vi "ArmKinematicsSimulator.vi"() -> ()   [LabVIEW 2020]
doc: "Simulates the inverse and forward kinematics for the configured robot arm on the computer, without needing to deploy to the robot."
uses:
  <vilib>/Utility/miscctls.llb/LV3DPointTypeDef.ctl
  GlobalArm.vi
  <vilib>/picture/3D Picture Control/Object/Create Object (drawable).vi
  <vilib>/picture/3D Picture Control/Object/Add Object (no reference).vi
  <vilib>/picture/3D Picture Control/NI_3D Picture Control.lvlib
  <vilib>/robotics/Kinematics/Plotting/NI_Robotics_3DKinematics.lvlib
panel:
  out "Wrist Power [-1, 1]":dbl format="%.2f"
  out "Elbow Power [-1. 1]":dbl format="%.2f"
  out "Shoulder Power [-1, 1]":dbl format="%.2f"
  in  "Intial Joint Angle Guesses (deg)":cluster{dbl, dbl, dbl}={90.0, 135.0, 0.0}
  in  "Goal End Effector Position":cluster{dbl, dbl, dbl}={180.0, -30.0, 25.0}
  in  "Reset 3D View":bool
  out "3D Arm Simulation":refnum<vi>(3d-picture)
  # "Pitch (deg)"
  # "X (in)"
  # "Z (in)"
  # "Shoulder (deg)"
  # "Elbow (deg)"
  # "Wrist (deg)"
  # "<-- DOWN FIELD              SCORING GRID -->"
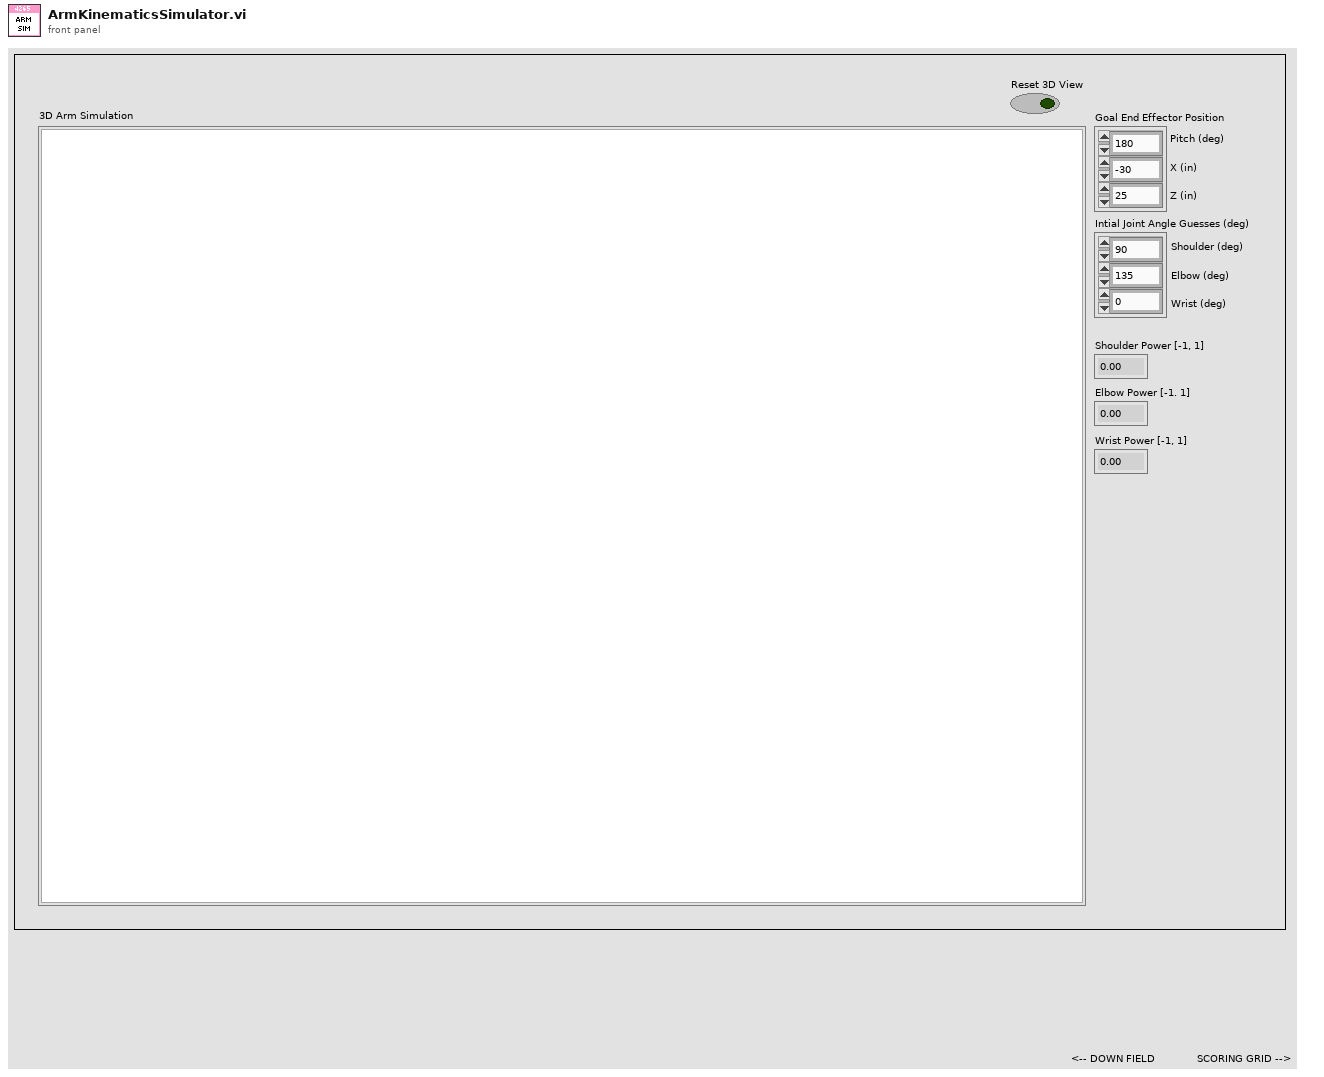
[diagram p1: front panel]
types:
  T1 = cluster{"Red":sgl, "Green":sgl, "Blue":sgl, "Alpha":sgl}
  T2 = typedef "LV3DPointTypeDef.ctl" = cluster{"X":sgl, "Y":sgl, "Z":sgl}
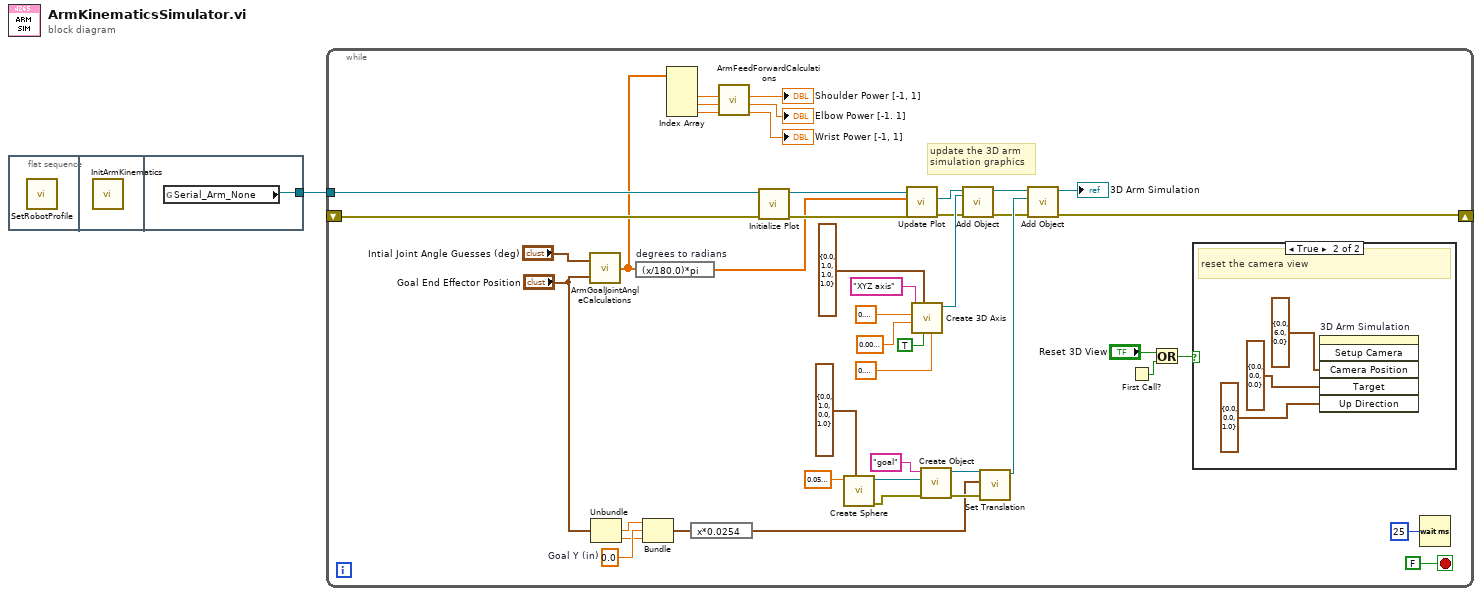
[diagram p0: block diagram]
diagram:
  n1 = flat-sequence {
    tunnel: [w2] -> w1
    frame #0 {
      n2 = call "SetRobotProfile.vi"() -> ()  [unwired: 1 in]
    }
    frame #1 {
      n3 = call "InitArmKinematics.vi"() -> ()  [unwired: 1 in]
    }
    frame #2 {
      n4 = global read "GlobalArm.vi" "Serial_Arm_None"() -> (w2:refnum<class "NI_Robotics_Serial Robot Arm.lvclass">)
    }
  }
  n5 = while {
    tunnel: w1 -> [w31]
    shift-right: [w22] -> _
    shift-left: _ -> [w30]
    stop <- FALSE stop-if-true
    w20 = 0.0  # Goal Y (in)
    # "update the 3D arm\nsimulation graphics"
    n6 = call "ArmGoalJointAngleCalculations.vi"("Goal End Effector Position"="Goal End Effector Position", "Intial Joint Angle Guesses (deg)"="Intial Joint Angle Guesses (deg)") -> ("Goal Joint Angles (deg)"=w9:dbl[])
    n7 = Unbundle("Goal End Effector Position") -> (w14:dbl, w13:dbl)  [unwired: 1 out]
    n8 = expression code="(x/180.0)*pi" "degrees to radians"(w9) -> (w16:dbl[])
    n9 = Bundle(w14, "Goal Y (in)"=w20, w13) -> (w19:cluster{dbl, "Goal Y (in)":dbl, dbl})  [unwired: 1 in]
    n10 = Index Array(array=w9) -> (element #2=w8:dbl, element #3=w7:dbl, element #4=w6:dbl)  [unwired: 4 in, 1 out]
    n11 = expression code="x*0.0254" ("degrees to radians")(w19) -> (w18:cluster{dbl, "Goal Y (in)":dbl, dbl})
    n12 = call "ArmFeedForwardCalculations.vi"("Wrist Pos (deg)"=w6, "Elbow Pos (deg)"=w7, "Shoulder Pos (deg)"=w8) -> ("Wrist Power [-1, 1]"=→"Wrist Power [-1, 1]":dbl, "Elbow Power [-1. 1]"=→"Elbow Power [-1. 1]":dbl, "Shoulder Power [-1, 1]"=→"Shoulder Power [-1, 1]":dbl)  [unwired: 6 in]
    n13 = call <vilib>:"Initialize Plot.vi"("error in (no error)"=w30, "serial arm in"=w31) -> ("error out"=w26:errorcluster, "serial arm out"=w25:refnum<class "NI_Robotics_Serial Robot Arm.lvclass">)  [unwired: 8 in]
    n14 = call <vilib>:"Create Sphere.vi"("Color"=T1 {"Red"=0.0, "Green"=1.0, "Blue"=0.0, "Alpha"=1.0}, "Radius"=sgl 0.05) -> ("error out"=w21:errorcluster, "New Sphere Refnum"=w27:refnum<vi>)  [unwired: 8 in]
    n15 = call <vilib>:"Update Plot.vi"("error in (no error)"=w26, "joint positions"=w16, "serial arm in"=w25) -> ("error out"=w24:errorcluster, "serial arm scene"=w45:refnum<vi>)  [unwired: 6 in, 1 out]
    n16 = call <vilib>:"Create 3D Axis.vi"("Character Size"=sgl 0.1, "Axis label?"=TRUE, "Color"=T1 {"Red"=0.0, "Green"=1.0, "Blue"=1.0, "Alpha"=1.0}, "Radius"=sgl 0.01, "Length"=sgl 0.2, "Name"="XYZ axis") -> ("New Object Refnum"=w38:refnum<vi>)  [unwired: 4 in, 1 out]
    n17 = call-poly <vilib>:"Create Object.vi"("error in (no error)"=w21, "Geometry"=w27, "Name"="goal") -> ("error out"=w35:errorcluster, "Scene:New Object"=w32:refnum<vi>)  [unwired: 7 in]
    n18 = call-poly <vilib>:"Add Object.vi"("error in (no error)"=w24, "New Object In"=w38, "Scene Object In"=w45) -> ("error out"=w23:errorcluster, "Scene Object Out"=w37:refnum<vi>)  [unwired: 7 in]
    n19 = call <vilib>:"Set Translation.vi"("error in (no error)"=w35, "Translation"=w18, "Scene Object"=w32) -> ("Translated Object"=w36:refnum<vi>)  [unwired: 7 in, 1 out]
    n20 = call-poly <vilib>:"Add Object.vi"("error in (no error)"=w23, "New Object In"=w36, "Scene Object In"=w37) -> ("error out"=w22:errorcluster, "Scene Object Out"=→"3D Arm Simulation":refnum<vi>)  [unwired: 7 in]
    n21 = First Call?() -> (First Call?: T/F=w12:bool)
    n22 = Or(x="Reset 3D View", y=w12) -> (x .or. y?=w11:bool)
    n23 = case shown="True" w11 {
      frame False {
      }
      frame True {
        # "reset the camera view"
        n24 = invoke on="3D Arm Simulation" class="SceneGraphDisp (strict)" method="Setup Camera"("Camera Position"=T2 {"X"=0.0, "Y"=6.0, "Z"=0.0}, "Target"=T2 {"X"=0.0, "Y"=0.0, "Z"=0.0}, "Up Direction"=T2 {"X"=0.0, "Y"=0.0, "Z"=1.0}) -> ()  [unwired: 3 in, 6 out]
      }
    }
    n25 = Wait (ms)(milliseconds to wait=u32 25) -> ()  [unwired: 1 out]
  }
